vi "Step Move Y.vi"(2 "Error In":errorcluster, 3 "Direction":bool=TRUE, 4 "No. of Y Steps":string="0", 5 "Reference In":refnum<class "_Controller.lvclass">) -> (0 "Error Out":errorcluster, 1 "Reference Out":refnum<class "_Controller.lvclass">)   [LabVIEW 2020]
doc: "Moves the XYZ scanning machine in the Y-direction. \n\nArgs:\n\nReference In: Incoming communication (reference) between LabView and the scanning rig controller\nError In: Checks for any errors with the incoming communication (reference)\nNo. of Y Steps: Number of steps the motor needs to move\nDirection: Boolean to control the direction the motor moves in \n\nReturns: \n\nReference Out: Output communnication (reference) between LabView and controller\nError Out: Checks for any error with output communication (reference)"
uses:
  <instrlib>/Arcus Ethernet Driver 1.0.0/ArcusEthernetComm/classes/Controller/_Controller.lvclass
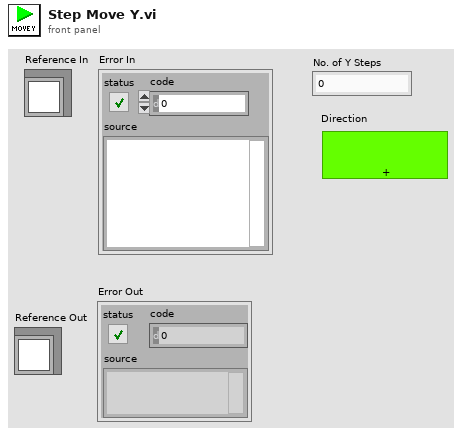
[diagram p1: front panel]
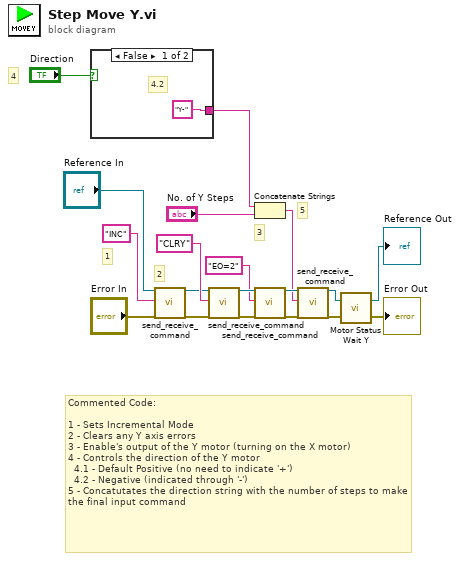
[diagram p0: block diagram]
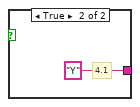
[diagram p2: hidden frame]
diagram:
  # "Commented Code:\n\n1 - Sets Incremental Mode \n2 - Clears any Y axis errors\n3 - Enable's output of the Y motor (turning on the X motor)\n4 - Controls the direction of the Y motor\n  4.1 - Default Positive (no need to indicate '+')\n  4.2 - Negative (indicated through '-') \n5 - Concatutates the direction string with the number of steps to make the final input command"
  # "5"
  # "4"
  # "3"
  # "2"
  # "1"
  n1 = case shown="False" "Direction" {
    tunnel: ["Y-" ("string") "Y" ("string")] -> w6
    frame False {
      # "4.2"
    }
    frame True {
      # "4.1"
    }
  }
  n2 = call <instrlib>:"send_receive_command.vi"("reference (in)"="Reference In", "ASCII Command (in)"="INC", "error in (no error)"="Error In") -> ("reference (out)"=w11:refnum<class "_Controller.lvclass">, "error out"=w8:errorcluster)  [unwired: 12 in, 3 out]
  n3 = call <instrlib>:"send_receive_command.vi"("reference (in)"=w11, "ASCII Command (in)"="CLRY", "error in (no error)"=w8) -> ("reference (out)"=w17:refnum<class "_Controller.lvclass">, "error out"=w18:errorcluster)  [unwired: 12 in, 3 out]
  n4 = Concatenate Strings(w6, "No. of Y Steps") -> (w14:string)
  n5 = call <instrlib>:"send_receive_command.vi"("reference (in)"=w17, "ASCII Command (in)"="EO=2", "error in (no error)"=w18) -> ("reference (out)"=w15:refnum<class "_Controller.lvclass">, "error out"=w16:errorcluster)  [unwired: 12 in, 3 out]
  n6 = call <instrlib>:"send_receive_command.vi"("reference (in)"=w15, "ASCII Command (in)"=w14, "error in (no error)"=w16) -> ("reference (out)"=w5:refnum<class "_Controller.lvclass">, "error out"=w4:errorcluster)  [unwired: 12 in, 3 out]
  n7 = call "Motor Status Wait Y.vi"("Error In"=w4, "Reference In"=w5) -> ("Error Out"=→"Error Out":errorcluster, "Reference Out"=→"Reference Out":refnum<class "_Controller.lvclass">)
